vi "Write Msg Input.vi"(10 "Msg Input":refnum<class "Msg Input.lvclass">, 11 "Stop Msg in":refnum<class "--Stop Msg.lvclass">) -> (3 "Stop Msg out":refnum<class "--Stop Msg.lvclass">)   [LabVIEW 2025, in "jettl.lvlib" / "Stop jettl Msg.lvlib" / "--Stop Msg.lvclass"]
uses:
  --Stop Msg.lvclass
  Msg Input/Msg Input.lvclass
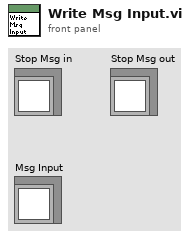
[diagram p1: front panel]
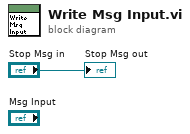
[diagram p0: block diagram]
diagram:
  "Stop Msg out" <- "Stop Msg in"
